vi "Open camera.vi"(8 "error in":errorcluster) -> (0 "error out":errorcluster, 3 "camera handle":i16)   [LabVIEW 2012]
uses:
  Visual Studio/Cascade wrapper/Release/Cascade wrapper.dll
panel:
  out "bitdepth":i16
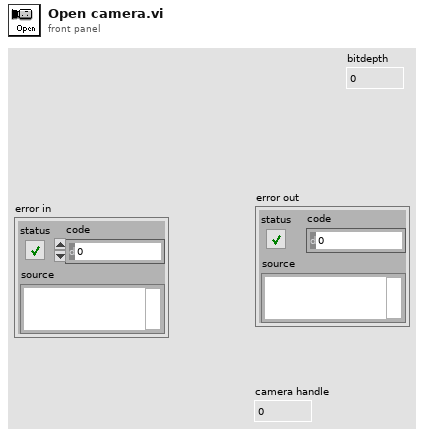
[diagram p1: front panel]
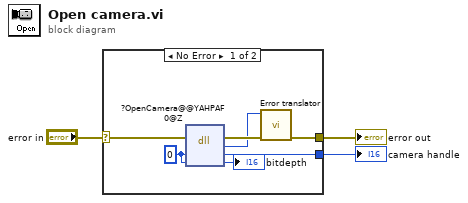
[diagram p0: block diagram]
diagram:
  n1 = case shown="No Error" "error in" {
    selector: "error in" -> [w10 w11]
    tunnel: [w7 w11] -> w2
    tunnel: [w9 _] -> w1
    frame No Error {
      w5 = i16 0 ("handle")
      n2 = dll-call lib="C:/moroder/Cascade wrapper/Visual Studio/Cascade wrapper/Release/Cascade wrapper.dll" fn="?OpenCamera@@YAHPAF0@Z"(error in=w10, "handle"=w5, "bitdepth"=w5) -> (error out=w8:errorcluster, "error"=w6:i32, "handle"=w9:i16, "bitdepth"=→"bitdepth":i16)  [unwired: 2 in, 1 out]
      n3 = call "Error translator.vi"("error in (no error)"=w8, "error code"=w6) -> ("error out"=w7:errorcluster)  [unwired: 9 in]
    }
    frame Error {
    }
  }
  "error out" <- w2
  "camera handle" <- w1
